vi "SourceNotifier.vi"(4 "Intensity":i32, 5 "Source":string, 6 "error in (no error)":errorcluster) -> (0 "error out":errorcluster)   [LabVIEW 2009]
uses:
  Controls/SourceStatus.ctl
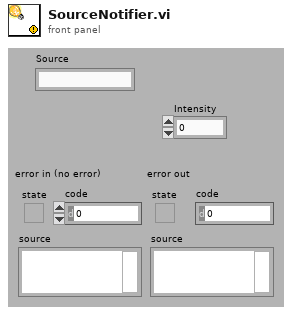
[diagram p1: front panel]
types:
  T1 = typedef "SourceStatus.ctl" = cluster{"Managed?":bool, "Intensity":i32}
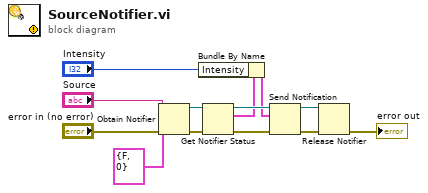
[diagram p0: block diagram]
diagram:
  n1 = Obtain Notifier(name (unnamed)="Source", notification data type=T1 {"Managed?"=FALSE, "Intensity"=0} ("SourceStatus"), error in (no error)="error in (no error)") -> (notifier out=w12:refnum<notifier>, error out=w1:errorcluster)  [unwired: 1 in, 1 out]
  n2 = Get Notifier Status(notifier=w12, error in (no error)=w1) -> (notifier out=w11:refnum<notifier>, current notification=w9:T1, error out=w10:errorcluster)  [unwired: 2 out]
  n3 = Bundle By Name(cluster=w9, "Intensity"="Intensity") -> (w8:T1)
  n4 = Send Notification(notification=w8, notifier=w11, error in (no error)=w10) -> (notifier out=w6:refnum<notifier>, error out=w7:errorcluster)
  n5 = Release Notifier(notifier=w6, error in (no error)=w7) -> (error out=→"error out":errorcluster)  [unwired: 3 out]
